vi "Memory.Pointer.U8.Dispose.vi"(8 "error in (no error)":errorcluster, 11 "U8 Pointer":refnum<class "Memory.Pointer.U8.lvclass">) -> (0 "error out":errorcluster)   [LabVIEW 2016, in "Memory.Pointer.U8.lvclass"]
doc: "Deallocates the block of memory represented by <b>Pointer</b>.\n\n<b>Warning</b>: This renders <b>Pointer</b> an invalid pointer. Any further attempts to access <b>Pointer</b> will cause a segfault (crash LabVIEW)."
uses:
  Memory.Pointer.U8.lvclass
  Pointer.Void/Memory.Pointer.Void.lvclass
  C:/Users/Ryan/Documents/Git/Sourcetree/LabVIEW-Memory-Manager/Source/Library/Classes/Pointer/Pointer.Numeric/Memory.Pointer.Numeric.lvclass
  C:/Users/Ryan/Documents/Git/Sourcetree/LabVIEW-Memory-Manager/Source/Library/Classes/Pointer/Pointer.Void/Memory.Pointer.Void.lvclass
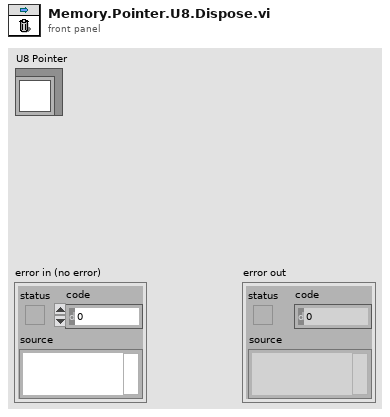
[diagram p1: front panel]
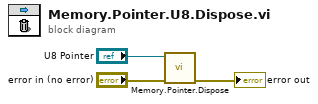
[diagram p0: block diagram]
diagram:
  n1 = call "Memory.Pointer.Dispose.vi"("error in (no error)"="error in (no error)", "Pointer in"="U8 Pointer") -> ("error out"=→"error out":errorcluster)  [unwired: 9 in]
